vi "Release All Message Queues.vi"(8 "error in (no error)":errorcluster, 11 "Message Queues":T1) -> (0 "error out":errorcluster)   [LabVIEW 2023, in "HAF.lvlib"]
doc: "Destroys all Message Queues, invalidating references and removing any existing messages on the queue."
uses:
  HAF.lvlib
  Message.ctl
  All Message Queues.ctl
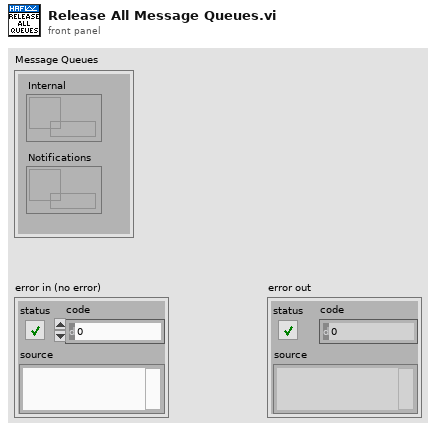
[diagram p1: front panel]
types:
  T1 = typedef "HAF.lvlib/All Message Queues.ctl" = cluster{"Internal":refnum<queue>, "Notifications":refnum<queue>}
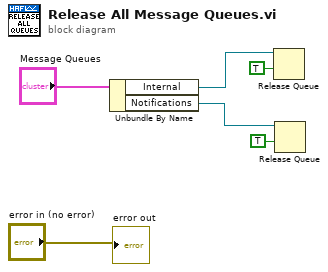
[diagram p0: block diagram]
diagram:
  n1 = Unbundle By Name("Message Queues") -> ("Internal"=w5:refnum<queue>, "Notifications"=w3:refnum<queue>)
  n2 = Release Queue(queue=w5, force destroy? (F)=TRUE) -> ()  [unwired: 1 in, 3 out]
  n3 = Release Queue(queue=w3, force destroy? (F)=TRUE) -> ()  [unwired: 1 in, 3 out]
  "error out" <- "error in (no error)"
